vi "Serial_Receive.vi"(8 "error in (no error)":errorcluster, 9 "timeoutMs":u32=100, 10 "Message ID":u32 format="%.0x", 11 "VISA resource name":refnum<visa-resource-name>) -> (0 "error out":errorcluster, 1 "data":u8[](array[numeric]), 2 "Message ID Out":u32 format="%x", 3 "VISA resource name out":refnum<visa-resource-name>)   [LabVIEW 2009, in "Serial.lvlib"]
doc: "Receives message from the serial port. To be used instead of CAN Receive VI from CAN for Jaguar FRC library"
uses:
  Serial.lvlib
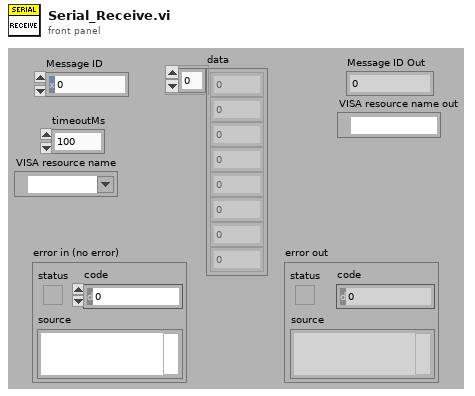
[diagram p1: front panel]
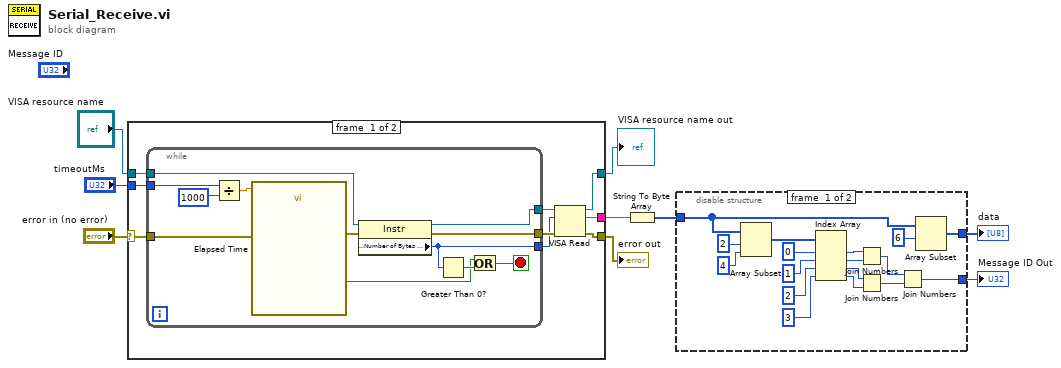
[diagram p0: block diagram]
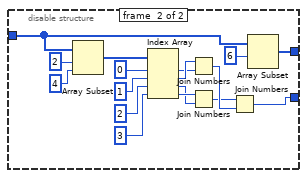
[diagram p2: hidden frame]
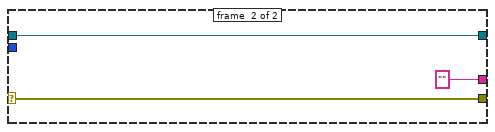
[diagram p3: hidden frame]
diagram:
  n1 = case shown="No Error" "error in (no error)" {
    selector: "error in (no error)" -> [w16 w32]
    tunnel: "timeoutMs" -> [w18 _]
    tunnel: [w14 w33] -> w3
    tunnel: "VISA resource name" -> [w17 w33]
    tunnel: [w12 w32] -> w2
    tunnel: [w10 "" ("read buffer")] -> w1
    frame #0 {
      n2 = while {
        tunnel: w18 -> [w21]
        tunnel: w16 -> [w24]
        tunnel: [w30] -> w13
        tunnel: [w27] -> w11
        tunnel: [w26] -> w15
        tunnel: w17 -> [w25]
        stop <- w29 stop-if-true
        n3 = Divide(x=w21, y=u32 1000) -> (x/y=w19:dbl)
        n4 = call "Elapsed Time"("Time Target (s)"=w19, "error in (no error)"=w24) -> ("Time has Elapsed"=w22:bool, "error out"=w23:errorcluster)  [unwired: 10 in, 6 out]
        n5 = property class="Instr"(reference=w25, error in=w23) -> (reference out=w26:refnum<visa-resource-name>, error out=w30:errorcluster, "Serial Settings:Number of Bytes at Serial Port"=w27:u32)
        n6 = Greater Than 0?(x=w27) -> (x > 0?=w28:bool)
        n7 = Or(x=w22, y=w28) -> (x .or. y?=w29:bool)
      }
      n8 = VISA Read(VISA resource name=w15, byte count=w11, error in (no error)=w13) -> (VISA resource name out=w14:refnum<visa-resource-name>, read buffer=w10:string, error out=w12:errorcluster)  [unwired: 1 out]
    }
    frame #1 {
    }
  }
  "error out" <- w2
  "VISA resource name out" <- w3
  n9 = String To Byte Array(string=w1) -> (unsigned byte array=w6:u8[])
  n10 = disable-structure shown="Enabled" {
    disable-tunnel: [w50 w56] -> w7
    disable-tunnel: w6 -> [w48 w57]
    disable-tunnel: [w45 w55] -> w5
    frame #0 {
      n11 = Array Subset(array=w48, index=2, length=4) -> (w42:u8[])
      n12 = Index Array(array=w42, index #1=0 ("index"), index #2=1 ("index"), index #3=2 ("index"), index #4=3 ("index")) -> (element #1=w37:u8, element #2=w36:u8, element #3=w35:u8, element #4=w34:u8)
      n13 = Join Numbers(hi=w37, lo=w36) -> ((hi.lo)=w44:u16)
      n14 = Join Numbers(hi=w35, lo=w34) -> ((hi.lo)=w43:u16)
      n15 = Join Numbers(hi=w44, lo=w43) -> ((hi.lo)=w45:u32)
      n16 = Array Subset(array=w48, index=6) -> (w50:u8[])  [unwired: 1 in]
    }
    frame #1 {
      n17 = Array Subset(array=w57, index=2, length=4) -> (w63:u8[])
      n18 = Index Array(array=w63, index #1=0 ("index"), index #2=1 ("index"), index #3=2 ("index"), index #4=3 ("index")) -> (element #1=w51:u8, element #2=w52:u8, element #3=w53:u8, element #4=w54:u8)
      n19 = Join Numbers(hi=w52, lo=w51) -> ((hi.lo)=w62:u16)
      n20 = Join Numbers(hi=w54, lo=w53) -> ((hi.lo)=w61:u16)
      n21 = Join Numbers(hi=w61, lo=w62) -> ((hi.lo)=w55:u32)
      n22 = Array Subset(array=w57, index=6) -> (w56:u8[])  [unwired: 1 in]
    }
  }
  "data" <- w7
  "Message ID Out" <- w5
